vi "Host Buffer and TDMS Status.vi"(4 "Read/Write Size (samples)":u32, 5 "Reset Max Count of TDMS Reads/Writes":bool, 6 "Initial Samples Transferred (0)":u64, 7 "Number of Pending Reads/Writes":u32, 9 "Reset Max Count of Elements Remaining":bool, 10 "Elements Remaining":u32, 11 "Elements In Region":u32) -> (1 "Host Buffer Status":cluster{u32, u32, u32}(slide)={0, 0, 2920792} scale=0.0..10000000.0 scale format="%#.1p", 2 "Samples Transferred":u64, 3 "Running Max of TDMS Reads/Writes":u32)   [LabVIEW 2013]
doc: "This SubVI Monitors the Host Side Buffer and the TDMS Writes. It returns Running Max of TDMS Reads/Writes, Samples Transfered from FPGA to Host, and the current status of the Host Side Buffer."
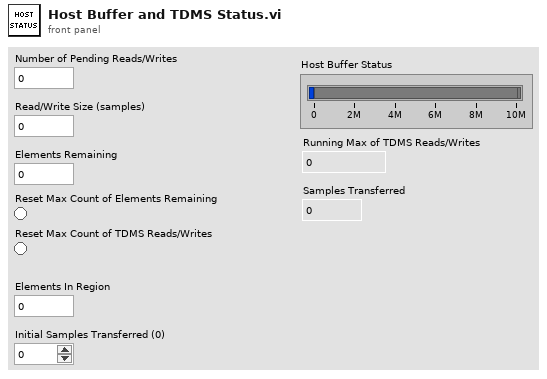
[diagram p1: front panel]
types:
  T1 = cluster{u32, "Elements Remaining":u32, "Running Max":u32}
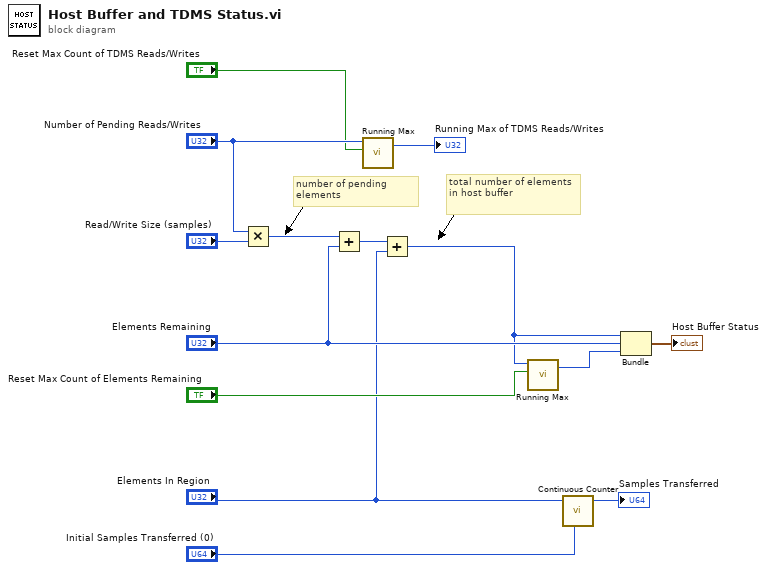
[diagram p0: block diagram]
diagram:
  # "number of pending elements"
  # "total number of elements in host buffer"
  n1 = Multiply(x="Number of Pending Reads/Writes", y="Read/Write Size (samples)") -> (x*y=w14:u32)
  n2 = Add(x=w14, y="Elements Remaining") -> (x+y=w4:u32)
  n3 = call "Running Max.vi"("Reset"="Reset Max Count of TDMS Reads/Writes", "Next Value"="Number of Pending Reads/Writes") -> ("Running Max"=→"Running Max of TDMS Reads/Writes":u32)  [unwired: 5 in]
  n4 = Add(x=w4, y="Elements In Region") -> (x+y=w2:u32)
  n5 = call "Running Max.vi"("Reset"="Reset Max Count of Elements Remaining", "Next Value"=w2) -> ("Running Max"=w6:u32)  [unwired: 5 in]
  n6 = call "Continuous Counter.vi"("value"="Elements In Region", "initial (0)"="Initial Samples Transferred (0)") -> ("count"=→"Samples Transferred":u64)  [unwired: 5 in]
  n7 = Bundle(w2, "Elements Remaining"="Elements Remaining", "Running Max"=w6) -> (→"Host Buffer Status":T1)  [unwired: 1 in]
